vi "Example Serial 2.vi"() -> ()   [LabVIEW 2018]
uses:
  Transcriptors/System API/Serial println string.vi
panel:
  out "Error Out":errorcluster
  in  "Error In":errorcluster
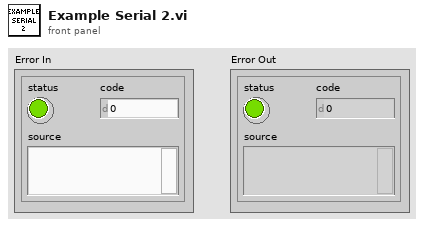
[diagram p1: front panel]
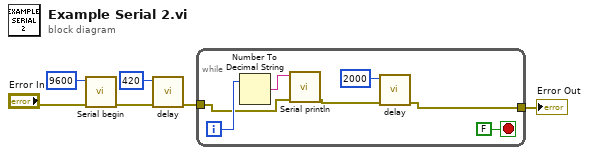
[diagram p0: block diagram]
diagram:
  n1 = call "Serial begin.vi"("Error In"="Error In", "speed (Bd)"=9600) -> ("Error Out"=w4:errorcluster)  [unwired: 9 in]
  n2 = call "delay.vi"("Error In"=w4, "time (ms)"=420) -> ("Error Out"=w2:errorcluster)  [unwired: 9 in]
  n3 = while {
    tunnel: w2 -> [w10]
    tunnel: [w7] -> w1
    i -> [w11]
    stop <- FALSE stop-if-true
    n4 = Number To Decimal String(number=w11) -> (decimal integer string=w12:string)  [unwired: 1 in]
    n5 = call-poly "Serial println.vi"("Error In"=w10, "string in"=w12) -> ("Error Out"=w8:errorcluster)  [unwired: 9 in]
    n6 = call "delay.vi"("Error In"=w8, "time (ms)"=2000) -> ("Error Out"=w7:errorcluster)  [unwired: 9 in]
  }
  "Error Out" <- w1
